vi "ROI entry screen-Generate user menu.vi"(11 "Functional Viewer Menu in":refnum<k9>) -> (0 "error out":errorcluster, 3 "Functional Viewer Menu":refnum<k9>)   [LabVIEW 2013]
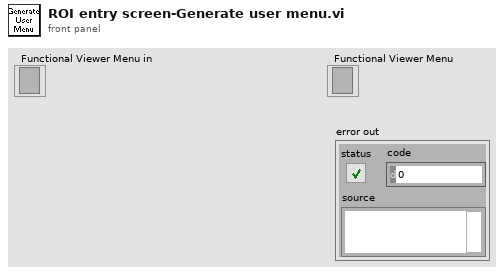
[diagram p1: front panel]
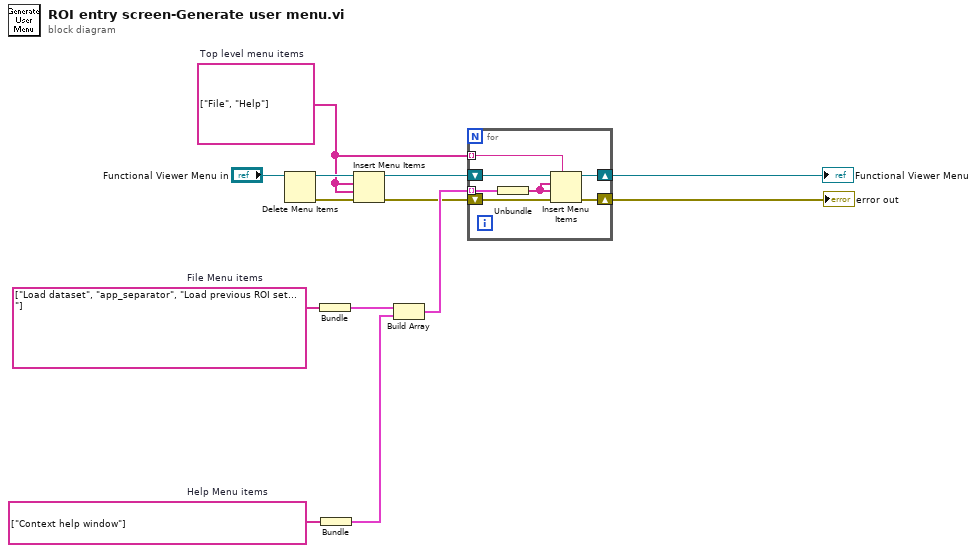
[diagram p0: block diagram]
diagram:
  w6 = string[] ["Context help window"]  # Help Menu items
  w8 = string[] ["Load dataset", "app_separator", "Load previous ROI set..."]  # File Menu items
  w9 = string[] ["File", "Help"]  # Top level menu items
  n1 = Delete Menu Items(9:"Functional Viewer Menu in") -> (0:w13:errorcluster, 3:w12:refnum<k9>)  [unwired: 3 in]
  n2 = Bundle("File Menu items"=w8) -> (w7:cluster{"File Menu items":string[]})  [unwired: 1 in]
  n3 = Bundle("Help Menu items"=w6) -> (w1:cluster{"Help Menu items":string[]})  [unwired: 1 in]
  n4 = Insert Menu Items(6:w13, 7:w9, 8:w9, 9:w12) -> (0:w2:errorcluster, 3:w10:refnum<k9>)  [unwired: 2 in, 1 out]
  n5 = Build Array(w7, w1) -> (w5:cluster{"Help Menu items":string[]}[])
  n6 = for {
    shift-right: [w19] -> w4
    shift-left: w10 -> [w20]
    tunnel: w9 -> [w18] mode=indexing
    tunnel: w5 -> [w17] mode=indexing
    shift-right: [w15] -> w3
    shift-left: w2 -> [w14]
    n7 = Unbundle(w17) -> ("Help Menu items"=w16:string[])
    n8 = Insert Menu Items(5:w18, 6:w14, 7:w16, 8:w16, 9:w20) -> (0:w15:errorcluster, 3:w19:refnum<k9>)  [unwired: 1 in, 1 out]
  }
  "error out" <- w3
  "Functional Viewer Menu" <- w4
